vi "comparenumber.vi"(9 "limit adjust":dbl, 10 "x":dbl, 11 "base":dbl) -> (1 "smaller":bool, 2 "equal":bool, 3 "bigger":bool)   [LabVIEW 2012]
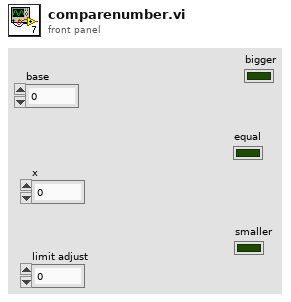
[diagram p1: front panel]
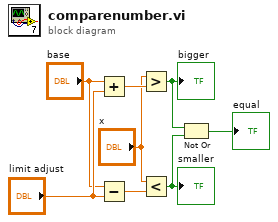
[diagram p0: block diagram]
diagram:
  n1 = Add(x="base", y="limit adjust") -> (x+y=w6:dbl)
  n2 = Subtract(x="base", y="limit adjust") -> (x-y=w7:dbl)
  n3 = Greater?(x="x", y=w6) -> (0:w5:bool)
  "bigger" <- w5
  n4 = Less?(x="x", y=w7) -> (x < y?=w4:bool)
  "smaller" <- w4
  n5 = Not Or(1:w4, 2:w5) -> (0:→"equal":bool)
